vi "CentroidBinning.vi"(7 "Settings.number of cam":dbl, 11 "spec cluster 3":cluster{"dp [MeV/C]":dbl[], dbl[]}[](graph)) -> (0 "spectrum":waveform(dbl), 1 "spec cluster":cluster{"xi used":dbl[], "yi":dbl[]}(graph), 2 "Charge [pC]":dbl format="%0.4f", 3 "specInfo":T1 {"Charge [pC]" format="%0.4f"}, 5 "time:specPost":u32)   [LabVIEW 2020]
uses:
  specInfo_TypDef.ctl
  <vilib>/Analysis/8numeric.llb/1D Numeric Integration.vi
  <vilib>/Analysis/1siggen.llb/Ramp Pattern by Delta.vi
  <vilib>/gmath/NI_Gmath.lvlib
  <vilib>/Analysis/NI_AALBase.lvlib
  <vilib>/Analysis/NI_AALPro.lvlib
  <vilib>/Analysis/NI_AAL_SigProc.lvlib
panel:
  out "spec cluster 2":cluster{dbl[], dbl[]}[](graph)
  out "peak energy (min)":dbl
  out "peak energy (max)":dbl
  out "mean":dbl
  out "fractional index or x":dbl
  out "max energy (10% of max counts)":dbl
  out "yi":dbl[](array[numeric]) format="%_6g"
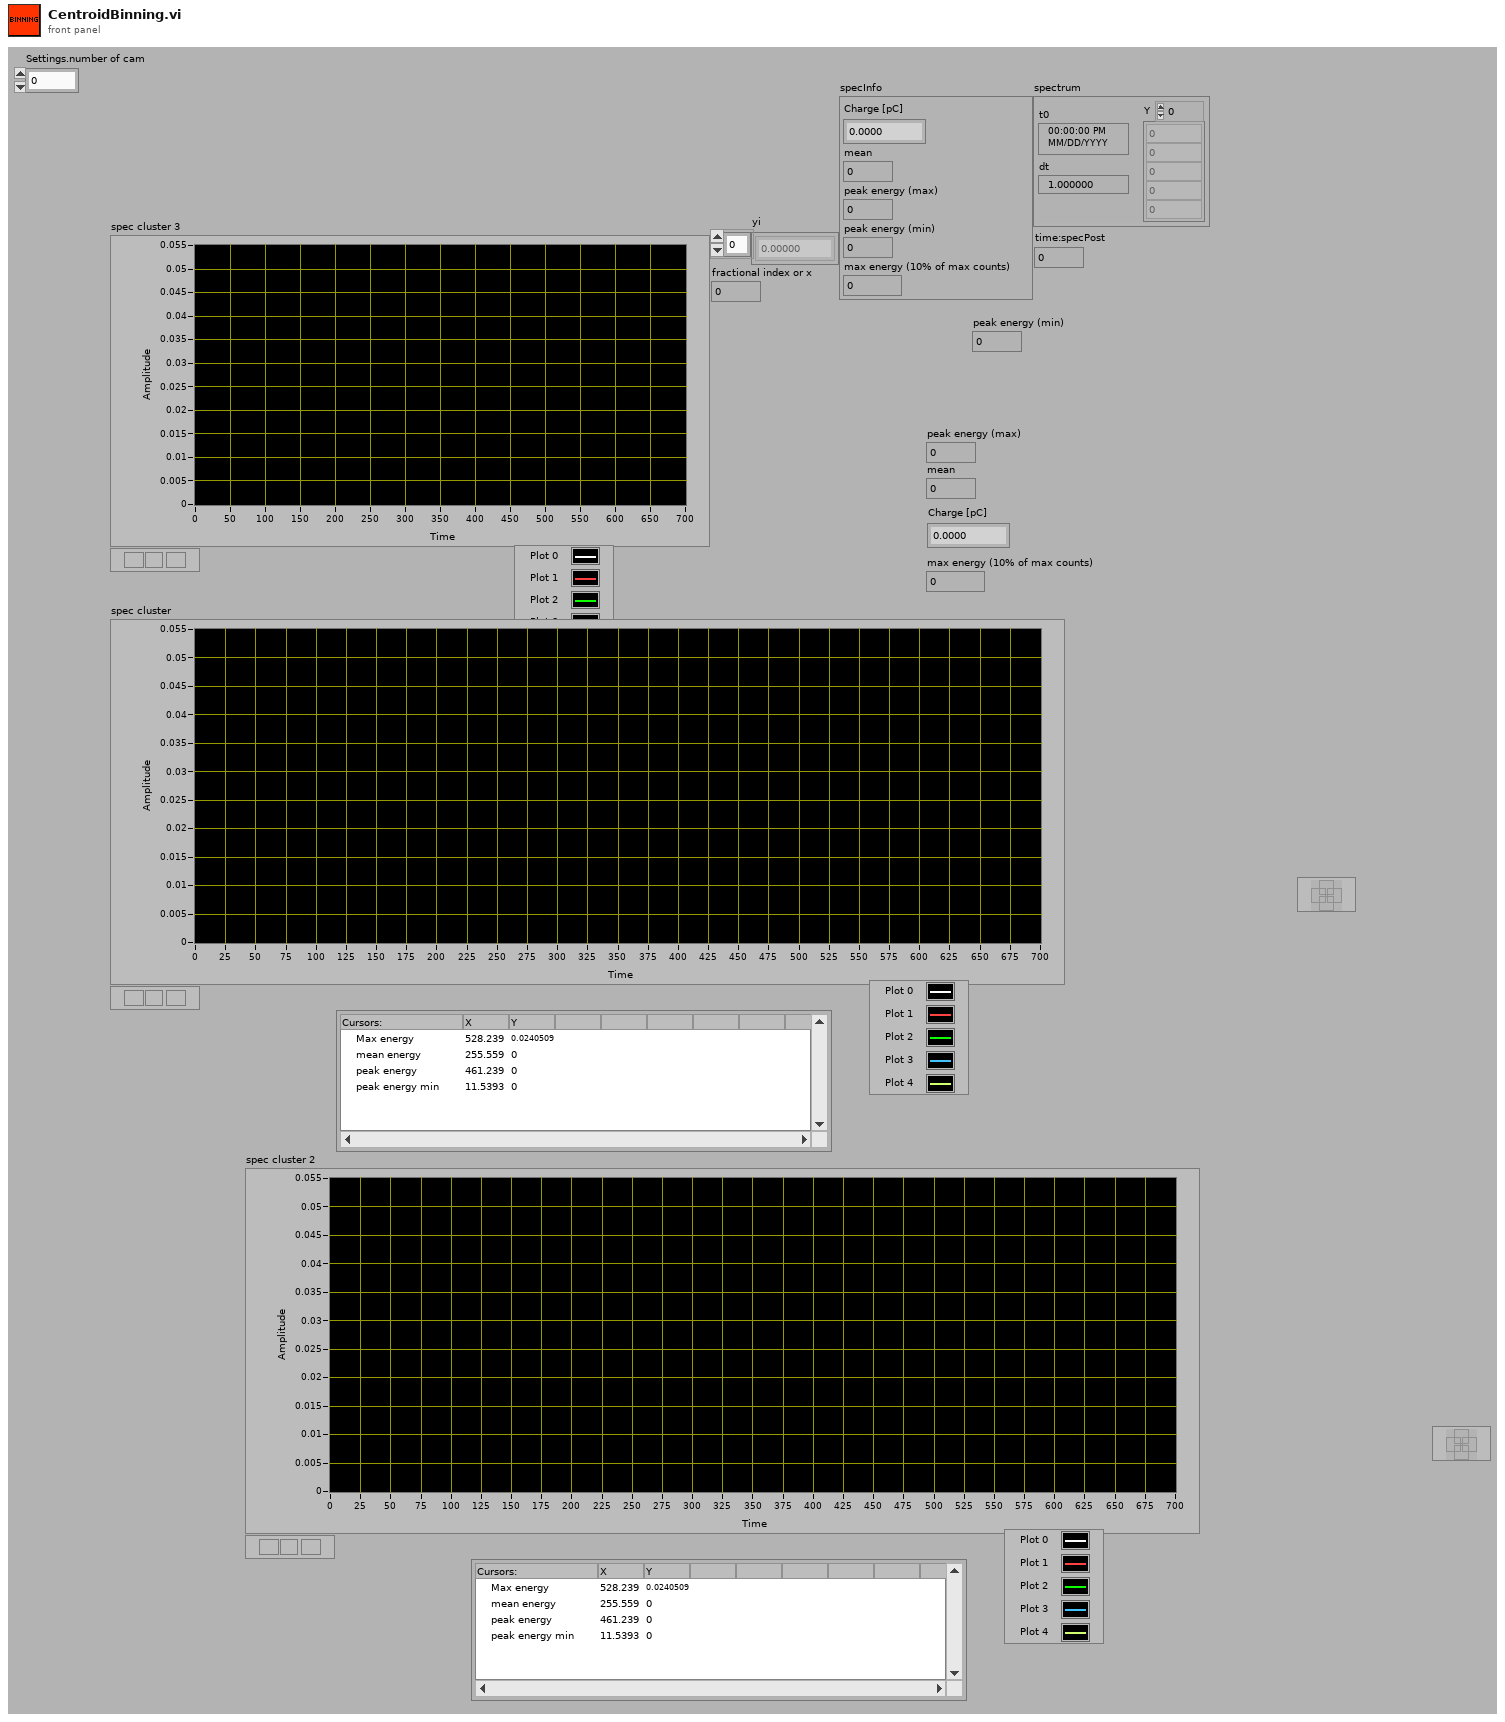
[diagram p1: front panel]
types:
  T1 = typedef "specInfo_TypDef.ctl" = cluster{"Charge [pC]":dbl, "mean":dbl, "peak energy (max)":dbl, "peak energy (min)":dbl, "max energy (10% of max counts)":dbl}
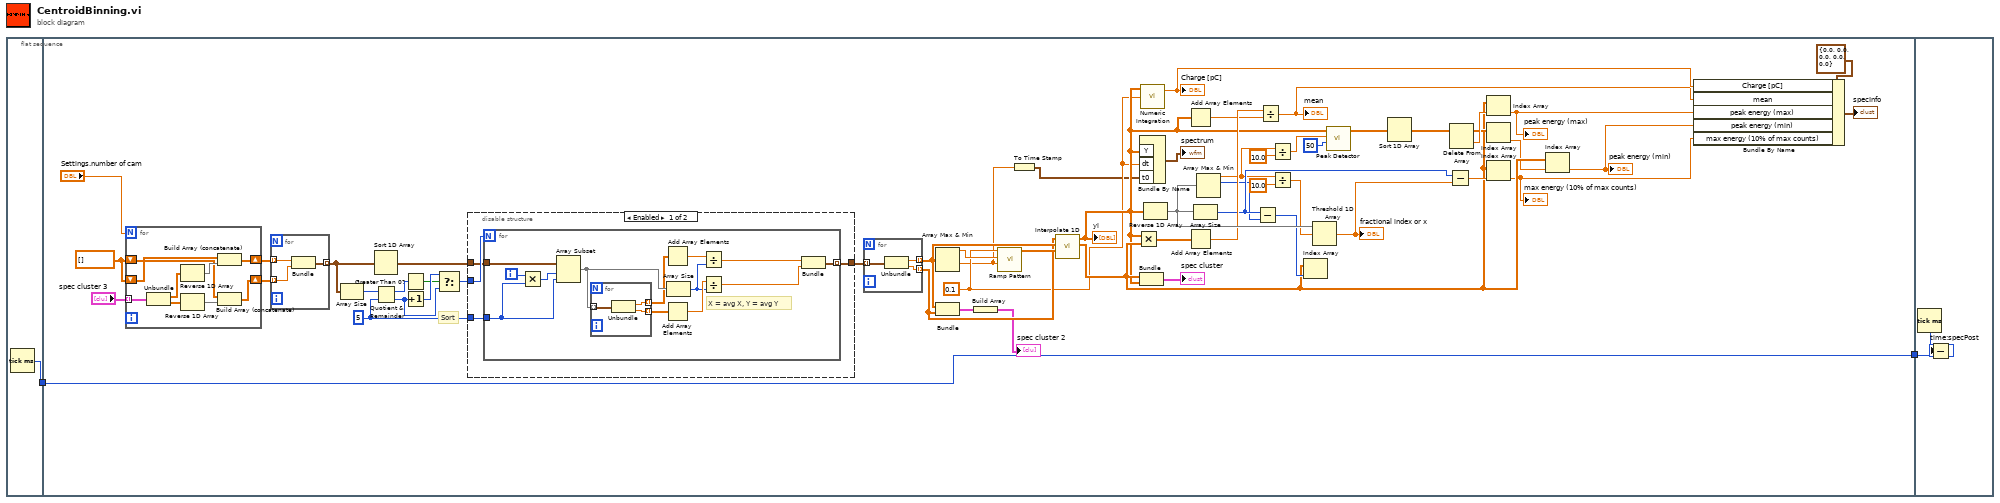
[diagram p0: block diagram]
diagram:
  n1 = flat-sequence {
    tunnel: [w3] -> w1
    tunnel: [w8] -> w2
    tunnel: w1 -> [w8]
    tunnel: w2 -> [w97]
    frame #0 {
      n2 = Tick Count (ms)() -> (millisecond timer value=w3:u32)
    }
    frame #1 {
      w10 = 0.1 ("delta")
      w48 = dbl[] []
      w55 = 5 ("Samples/bin")
      # "Sort"
      n3 = for {
        N: "Settings.number of cam" -> [_]
        tunnel: "spec cluster 3" -> [w89] mode=indexing
        shift-right: [w86] -> w47
        shift-left: w48 -> [w85]
        shift-right: [w82] -> w42
        shift-left: w48 -> [w81]
        n4 = Unbundle(w89) -> ("dp [MeV/C]"=w88:dbl[], w84:dbl[])
        n5 = Reverse 1D Array(array=w88) -> (reversed array=w87:dbl[])
        n6 = Reverse 1D Array(array=w84) -> (reversed array=w83:dbl[])
        n7 = Build Array (concatenate)(w85, w87) -> (w86:dbl[])
        n8 = Build Array (concatenate)(w81, w83) -> (w82:dbl[])
      }
      n9 = for {
        tunnel: w47 -> [w95] mode=indexing
        tunnel: w42 -> [w94] mode=indexing
        tunnel: [w93] -> w52 mode=indexing
        n10 = Bundle(w95, w94) -> (w93:cluster{dbl, dbl})  [unwired: 1 in]
      }
      n11 = Array Size(array=w52) -> (size(s)=w53:i32)
      n12 = Sort 1D Array(array=w52) -> (sorted array=w50:cluster{dbl, dbl}[])
      n13 = Quotient & Remainder(x=w53, y=w55) -> (x-y*floor(x/y)=w59:i32, floor(x/y)=w57:i32)
      n14 = Greater Than 0?(x=w59) -> (x > 0?=w56:bool)
      n15 = Increment(x=w57) -> (x+1=w58:i32)
      n16 = Select(t=w58, s=w56, f=w57) -> (s? t:f=w54:i32)
      n17 = disable-structure shown="Enabled" {
        disable-tunnel: w55 -> [w63 _]
        disable-tunnel: w54 -> [w62 _]
        disable-tunnel: [w61 w80] -> w51
        disable-tunnel: w50 -> [w60 w80]
        frame Enabled {
          n18 = for {
            N: w62 -> [_]
            tunnel: w60 -> [w76]
            tunnel: w63 -> [w74]
            tunnel: [w71] -> w61 mode=indexing
            i -> [w75]
            # "X = avg X, Y = avg Y"
            n19 = Multiply(x=w75, y=w74) -> (x*y=w73:i32)
            n20 = Array Subset(array=w76, index=w73, length=w74) -> (w72:cluster{dbl, dbl}[])
            n21 = for {
              tunnel: w72 -> [w79] mode=indexing
              tunnel: [w78] -> w70 mode=indexing
              tunnel: [w77] -> w69 mode=indexing
              n22 = Unbundle(w79) -> (w78:dbl, w77:dbl)
            }
            n23 = Add Array Elements(numeric array=w70) -> (sum=w67:dbl)
            n24 = Add Array Elements(numeric array=w69) -> (sum=w68:dbl)
            n25 = Array Size(array=w72) -> (size(s)=w66:i32)
            n26 = Divide(x=w67, y=w66) -> (x/y=w65:dbl)
            n27 = Divide(x=w68, y=w66) -> (x/y=w64:dbl)
            n28 = Bundle(w65, w64) -> (w71:cluster{dbl, dbl})  [unwired: 1 in]
          }
        }
        frame Disabled {
        }
      }
      n29 = for {
        tunnel: w51 -> [w92] mode=indexing
        tunnel: [w91] -> w44 mode=indexing
        tunnel: [w90] -> w43 mode=indexing
        n30 = Unbundle(w92) -> (w91:dbl, w90:dbl)
      }
      n31 = Array Max & Min(array=w44) -> (max value=w46:dbl, min value=w5:dbl)  [unwired: 2 out]
      n32 = Bundle(w44, w43) -> (w41:cluster{dbl[], dbl[]})  [unwired: 1 in]
      n33 = Build Array(w41) -> (→"spec cluster 2":cluster{dbl[], dbl[]}[])
      n34 = call-poly <vilib>:"Ramp Pattern.vi"("start"=w5, "end"=w46, "delta"=w10) -> ("Ramp Pattern"=w45:dbl[])  [unwired: 6 in, 2 out]
      n35 = To Time Stamp(1:w5) -> (0:w4:timestamp)
      n36 = call <vilib>:"Interpolate 1D.vi"("xi"=w45, "X"=w44, "Y"=w43) -> ("xi used"=w20:dbl[], "yi"=w11:dbl[])  [unwired: 6 in, 1 out]
      "yi" <- w11
      n37 = Multiply(x=w11, y=w20) -> (x*y=w34:dbl[])
      n38 = Bundle By Name("Y"=w11, "dt"=w10, "t0"=w4) -> (→"spectrum":waveform(dbl))  [unwired: 1 in]
      n39 = Bundle("xi used"=w20, "yi"=w11) -> (→"spec cluster":cluster{"xi used":dbl[], "yi":dbl[]})  [unwired: 1 in]
      n40 = call-poly <vilib>:"Numeric Integration.vi"("dt"=w10, "Input Array"=w11) -> ("result"=w17:dbl)  [unwired: 1 in, 1 out]
      "Charge [pC]" <- w17
      n41 = Reverse 1D Array(array=w11) -> (reversed array=w39:dbl[])
      n42 = Add Array Elements(numeric array=w11) -> (sum=w32:dbl)
      n43 = Add Array Elements(numeric array=w34) -> (sum=w33:dbl)
      n44 = Array Size(array=w39) -> (size(s)=w31:i32)
      n45 = Array Max & Min(array=w39) -> (max value=w28:dbl, max index (indices)=w30:i32)  [unwired: 2 out]
      n46 = Subtract(x=w31, y=w30) -> (x-y=w29:i32)
      n47 = Divide(x=w33, y=w32) -> (x/y=w16:dbl)
      "mean" <- w16
      n48 = Divide(x=w28, y=10.0) -> (x/y=w26:dbl)
      n49 = Divide(x=w28, y=10.0) -> (x/y=w35:dbl)
      n50 = Index Array(array=w20, index=w29) -> ()  [unwired: 1 out]
      n51 = Threshold 1D Array(2:w35, 3:w39) -> (0:w38:dbl)  [unwired: 1 in]
      "fractional index or x" <- w38
      n52 = call <vilib>:"Peak Detector.vi"("width"=50, "threshold"=w26, "X"=w11) -> ("Locations"=w24:dbl[])  [unwired: 4 in, 4 out]
      n53 = Sort 1D Array(array=w24) -> (sorted array=w23:dbl[])
      n54 = Subtract(x=w31, y=w38) -> (x-y=w36:dbl)
      n55 = Delete From Array(array=w23) -> (deleted portion=w22:dbl, array with subset deleted=w21:dbl[])  [unwired: 2 in]
      n56 = Index Array(array=w20, index=w22) -> (element=w15:dbl)
      "peak energy (max)" <- w15
      n57 = Index Array(array=w21) -> (element=w19:dbl)  [unwired: 1 in]
      n58 = Index Array(array=w20, index=w36) -> (element=w13:dbl)
      "max energy (10% of max counts)" <- w13
      n59 = Index Array(array=w20, index=w19) -> (element=w14:dbl)
      "peak energy (min)" <- w14
      n60 = Bundle By Name(cluster=T1 {"Charge [pC]"=0.0, "mean"=0.0, "peak energy (max)"=0.0, "peak energy (min)"=0.0, "max energy (10% of max counts)"=0.0} ("specInfo"), "Charge [pC]"=w17, "mean"=w16, "peak energy (max)"=w15, "peak energy (min)"=w14, "max energy (10% of max counts)"=w13) -> (→"specInfo":T1)
    }
    frame #2 {
      n61 = Tick Count (ms)() -> (millisecond timer value=w98:u32)
      n62 = Subtract(x=w98, y=w97) -> (x-y=→"time:specPost":u32)
    }
  }
